vi "Deallocate Multiple Blocks.vi"(8 "error in (no error)":errorcluster, 10 "Block Descriptors":T1[](array[typedef]) {"next descriptor ptr" format="%08x"; "data size" format="%08x"; "data ptr (upper)" format="%08x"; "data ptr (lower)" format="%08x"; "descriptor ptr (aligned)" format="%08x"; "descriptor size" format="%08x"; "descriptor ptr (VISA)" format="%08x"}, 11 "GE 5565PIORC in":refnum<class "GE 5565PIORC.lvclass">) -> (0 "error out":errorcluster, 3 "GE 5565PIORC out":refnum<class "GE 5565PIORC.lvclass">)   [LabVIEW 2016, in "GE 5565PIORC.lvclass"]
uses:
  GE 5565PIORC.lvclass
  Controls/DMA Block Descriptor.ctl
  GE 5565PIORC.lvclass/GE 5565PIORC.ctl
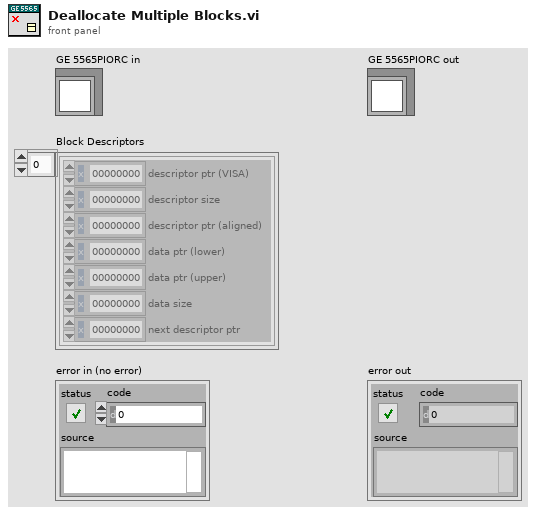
[diagram p1: front panel]
types:
  T1 = typedef "GE 5565PIORC.lvclass/DMA Block Descriptor.ctl" = cluster{"descriptor ptr (VISA)":u32, "descriptor size":u32, "descriptor ptr (aligned)":u32, "data ptr (lower)":u32, "data ptr (upper)":u32, "data size":u32, "next descriptor ptr":u32}
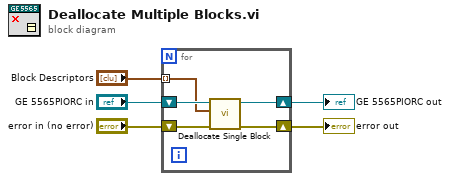
[diagram p0: block diagram]
diagram:
  n1 = for {
    shift-right: [w9] -> w4
    shift-left: "error in (no error)" -> [w10]
    shift-right: [w7] -> w2
    shift-left: "GE 5565PIORC in" -> [w8]
    tunnel: "Block Descriptors" -> [w6] mode=indexing
    n2 = call "Deallocate Single Block.vi"("error in (no error)"=w10, "Block Descriptor"=w6, "GE 5565PIORC in"=w8) -> ("error out"=w9:errorcluster, "GE 5565PIORC out"=w7:refnum<class "GE 5565PIORC.lvclass">)  [unwired: 7 in]
  }
  "error out" <- w4
  "GE 5565PIORC out" <- w2
